vi "ADIS16448 IMU Calibration.vi"() -> ()   [LabVIEW 2015]
uses:
  <vilib>/Rock Robotics/SystemInterfaces/spilib/spi_bus.ctl
  <vilib>/Rock Robotics/WPI/SPI/WPI_SPIDevRef.ctl
  ADI MXP IMU/WPI_IMU_ADIS16448_Registers.ctl
  ADI MXP IMU/FRC_ADIS16448_IMU.lvlib
panel:
  out "Offset Registers":T1 {"zGYRO_OFF" format="%x"; "yGYRO_OFF" format="%x"; "xGYRO_OFF" format="%x"}
  out "Write Successful?":bool
  out "Timer":i32
  out "Device Found":bool
  # "FRC Analog Devices ADIS16448 IMU\nOffset Calibration Program"
  # "Instructions: \n* Place your robot in a stable location where it will not be bumped or moved.\n* Make sure that the IMU is securely mounted to the RoboRIO! \n* When ready, start the VI. The program will enable averaging inside of the IMU and will calculate the bias offset. \n* After recording data, the VI will save the data within the sensor for future use. \n* Running this utility again will overwrite the bias correction ."
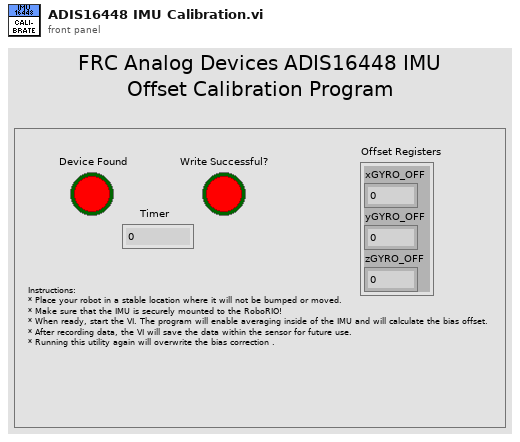
[diagram p1: front panel]
types:
  T1 = cluster{"xGYRO_OFF":u16, "yGYRO_OFF":u16, "zGYRO_OFF":u16}
  T2 = typedef "WPI_SPIDevRef.ctl" = cluster{"DevStatus":errorcluster, "Handle":i32, "SPI Bus":T3}
  T3 = typedef "spi_bus.ctl" = enum16{"SPI On-Board, CS0", "SPI On-Board, CS1", "SPI On-Board, CS2", "SPI On-Board, CS3", "SPI MXP", "Invalid"}
  T4 = typedef "FRC_ADIS16448_IMU.lvlib/WPI_IMU_ADIS16448_InterruptDevRef.ctl" = cluster{"ADI IMU DevRef":T5, "InterruptRef":T6}
  T5 = typedef "FRC_ADIS16448_IMU.lvlib/WPI_IMU_ADIS16448_IMUDevRef.ctl" = cluster{"DevStatus":errorcluster, "Handle":i32, "SPI Bus":T3, "Device Found":bool, "Device Ready":bool, "Yaw Axis":enum16{"X", "Y", "Z"}, "AHRS Algorithm":enum16{"Complementary", "Madgwick"}, "Serial":u16, "Lot ID 2":u16, "Lot ID 1":u16, "Product ID":u16}
  T6 = typedef "WPI_InterruptRef.ctl" = cluster{"DevStatus":errorcluster, "InterruptIndex":T7}
  T7 = typedef "FPGA_InterruptIndex.ctl" = enum8{"0", "1", "2", "3", "4", "5", "6", "7", "Invalid"}
  T8 = typedef "FRC_ADIS16448_IMU.lvlib/WPI_IMU_ADIS16448_Registers.ctl" = u8
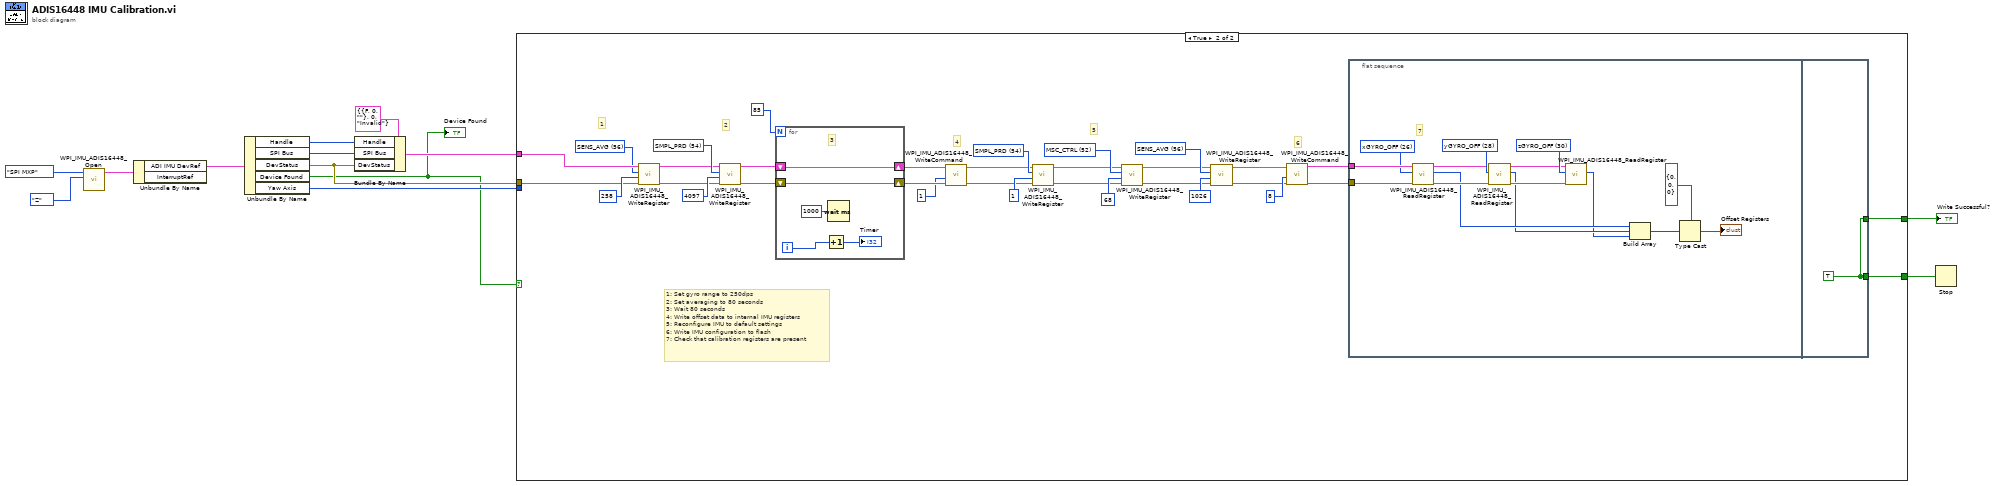
[diagram p0: block diagram]
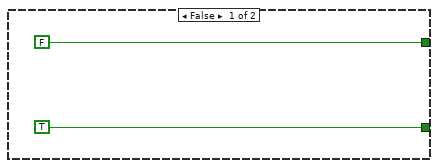
[diagram p2: hidden frame]
diagram:
  n1 = call "WPI_IMU_ADIS16448_Open.vi"("Yaw Axis"=enum16{"X", "Y", "Z"}."Z" ("Z Axis"), "SPI Chip Select"=spi_bus."SPI MXP") -> ("ADI IMU Interrupt DevRef"=w8:T4)  [unwired: 8 in, 1 out]
  n2 = Unbundle By Name(w8) -> ("ADI IMU DevRef"=w9:T5)  [unwired: 1 out]
  n3 = Unbundle By Name(w9) -> ("Handle"=w11:i32, "SPI Bus"=w10:T3, "DevStatus"=w5:errorcluster, "Device Found"=w1:bool, "Yaw Axis"=w6:enum16{"X", "Y", "Z"})
  "Device Found" <- w1
  n4 = Bundle By Name(cluster=T2 {"DevStatus"={"status"=FALSE, "code"=0, "source"=""}, "Handle"=0, "SPI Bus"=enum."Invalid"} ("SPIDevRef out"), "Handle"=w11, "SPI Bus"=w10, "DevStatus"=w5) -> (w7:T2)
  n5 = case shown="True" w1 {
    tunnel: w7 -> [_ w48]
    tunnel: w6 -> [_ _]
    tunnel: w5 -> [_ w45]
    tunnel: [TRUE w29] -> w3
    tunnel: [FALSE w16] -> w2
    frame False {
    }
    frame True {
      w32 = T8 56 items=["GLOB_CMD"=62, "SEQ_CNT"=58, "SMPL_PRD"=54, "SENS_AVG"=56, "MSC_CTRL"=52, "ERROR_FLAGS"=60, "TEMP"=44, "BARO"=40, "Z_MAG"=36, "Y_MAG"=32, "X_MAG"=28, "Z_ACCEL"=24, "Y_ACCEL"=20, "X_ACCEL"=16, "Z_GYRO"=12, "Y_GYRO"=8, "X_GYRO"=4, "PROD_ID"=86, "LOT_ID2"=84, "LOT_ID1"=82, "SERIAL_NUM"=88] ("ADIS16448 Register")
      w33 = T8 52 items=["GLOB_CMD"=62, "SEQ_CNT"=58, "SMPL_PRD"=54, "SENS_AVG"=56, "MSC_CTRL"=52, "ERROR_FLAGS"=60, "TEMP"=44, "BARO"=40, "Z_MAG"=36, "Y_MAG"=32, "X_MAG"=28, "Z_ACCEL"=24, "Y_ACCEL"=20, "X_ACCEL"=16, "Z_GYRO"=12, "Y_GYRO"=8, "X_GYRO"=4, "PROD_ID"=86, "LOT_ID2"=84, "LOT_ID1"=82, "SERIAL_NUM"=88] ("ADIS16448 Register")
      w31 = T8 54 items=["GLOB_CMD"=62, "SEQ_CNT"=58, "SMPL_PRD"=54, "SENS_AVG"=56, "MSC_CTRL"=52, "ERROR_FLAGS"=60, "TEMP"=44, "BARO"=40, "Z_MAG"=36, "Y_MAG"=32, "X_MAG"=28, "Z_ACCEL"=24, "Y_ACCEL"=20, "X_ACCEL"=16, "Z_GYRO"=12, "Y_GYRO"=8, "X_GYRO"=4, "PROD_ID"=86, "LOT_ID2"=84, "LOT_ID1"=82, "SERIAL_NUM"=88] ("ADIS16448 Register")
      w44 = T8 54 items=["GLOB_CMD"=62, "SEQ_CNT"=58, "SMPL_PRD"=54, "SENS_AVG"=56, "MSC_CTRL"=52, "ERROR_FLAGS"=60, "TEMP"=44, "BARO"=40, "Z_MAG"=36, "Y_MAG"=32, "X_MAG"=28, "Z_ACCEL"=24, "Y_ACCEL"=20, "X_ACCEL"=16, "Z_GYRO"=12, "Y_GYRO"=8, "X_GYRO"=4, "PROD_ID"=86, "LOT_ID2"=84, "LOT_ID1"=82, "SERIAL_NUM"=88] ("ADIS16448 Register")
      w47 = T8 56 items=["GLOB_CMD"=62, "SEQ_CNT"=58, "SMPL_PRD"=54, "SENS_AVG"=56, "MSC_CTRL"=52, "ERROR_FLAGS"=60, "TEMP"=44, "BARO"=40, "Z_MAG"=36, "Y_MAG"=32, "X_MAG"=28, "Z_ACCEL"=24, "Y_ACCEL"=20, "X_ACCEL"=16, "Z_GYRO"=12, "Y_GYRO"=8, "X_GYRO"=4, "PROD_ID"=86, "LOT_ID2"=84, "LOT_ID1"=82, "SERIAL_NUM"=88] ("ADIS16448 Register")
      # "5"
      # "6"
      # "4"
      # "2"
      # "1"
      # "1: Set gyro range to 250dps\n2: Set averaging to 80 seconds\n3: Wait 80 seconds\n4: Write offset data to internal IMU registers\n5: Reconfigure IMU to default settings\n6: Write IMU configuration to flash\n7: Check that calibration registers are present"
      n6 = call "WPI_IMU_ADIS16448_WriteRegister.vi"("error in (no error)"=w45, "Data"=u16 258, "ADIS16448 Register"=w47, "SPIDevRef in"=w48) -> ("error out"=w27:errorcluster, "SPIDevRef out"=w28:T2)  [unwired: 6 in]
      n7 = call "WPI_IMU_ADIS16448_WriteRegister.vi"("error in (no error)"=w27, "Data"=u16 4097, "ADIS16448 Register"=w44, "SPIDevRef in"=w28) -> ("error out"=w40:errorcluster, "SPIDevRef out"=w41:T2)  [unwired: 6 in]
      n8 = for {
        N: 85 -> [_]
        shift-right: [w68] -> w39
        shift-left: w41 -> [w68]
        shift-right: [w67] -> w38
        shift-left: w40 -> [w67]
        i -> [w65]
        # "3"
        n9 = Increment(x=w65) -> (x+1=→"Timer":i32)
        n10 = Wait (ms)(milliseconds to wait=u32 1000) -> ()  [unwired: 1 out]
      }
      n11 = call "WPI_IMU_ADIS16448_WriteCommand.vi"("error in (no error)"=w38, "Data"=u16 1, "SPIDevRef in"=w39) -> ("error out"=w25:errorcluster, "SPIDevRef out"=w26:T2)  [unwired: 7 in]
      n12 = call "WPI_IMU_ADIS16448_WriteRegister.vi"("error in (no error)"=w25, "Data"=u16 1, "ADIS16448 Register"=w31, "SPIDevRef in"=w26) -> ("error out"=w21:errorcluster, "SPIDevRef out"=w22:T2)  [unwired: 6 in]
      n13 = call "WPI_IMU_ADIS16448_WriteRegister.vi"("error in (no error)"=w21, "Data"=u16 68, "ADIS16448 Register"=w33, "SPIDevRef in"=w22) -> ("error out"=w23:errorcluster, "SPIDevRef out"=w24:T2)  [unwired: 6 in]
      n14 = call "WPI_IMU_ADIS16448_WriteRegister.vi"("error in (no error)"=w23, "Data"=u16 1026, "ADIS16448 Register"=w32, "SPIDevRef in"=w24) -> ("error out"=w19:errorcluster, "SPIDevRef out"=w20:T2)  [unwired: 6 in]
      n15 = call "WPI_IMU_ADIS16448_WriteCommand.vi"("error in (no error)"=w19, "Data"=u16 8, "SPIDevRef in"=w20) -> ("error out"=w17:errorcluster, "SPIDevRef out"=w18:T2)  [unwired: 7 in]
      n16 = flat-sequence {
        tunnel: w18 -> [w63]
        tunnel: w17 -> [w62]
        tunnel: [w64] -> w29
        tunnel: [w64] -> w16
        frame #0 {
          w59 = T8 30 items=["zGYRO_OFF"=30, "yGYRO_OFF"=28, "xGYRO_OFF"=26, "GLOB_CMD"=62, "SEQ_CNT"=58, "SMPL_PRD"=54, "SENS_AVG"=56, "MSC_CTRL"=52, "zACCEL_OFF"=36, "yACCEL_OFF"=34, "xACCEL_OFF"=32, "ERROR_FLAGS"=60, "TEMP"=24, "BARO"=22, "Z_MAG"=20, "Y_MAG"=18, "X_MAG"=16, "Z_ACCEL"=14, "Y_ACCEL"=12, "X_ACCEL"=10, "Z_GYRO"=8, "Y_GYRO"=6, "X_GYRO"=4, "PROD_ID"=86, "LOT_ID2"=84, "LOT_ID1"=82, "SERIAL_NUM"=88] ("ADIS16448 Register")
          w60 = T8 28 items=["zGYRO_OFF"=30, "yGYRO_OFF"=28, "xGYRO_OFF"=26, "GLOB_CMD"=62, "SEQ_CNT"=58, "SMPL_PRD"=54, "SENS_AVG"=56, "MSC_CTRL"=52, "zACCEL_OFF"=36, "yACCEL_OFF"=34, "xACCEL_OFF"=32, "ERROR_FLAGS"=60, "TEMP"=24, "BARO"=22, "Z_MAG"=20, "Y_MAG"=18, "X_MAG"=16, "Z_ACCEL"=14, "Y_ACCEL"=12, "X_ACCEL"=10, "Z_GYRO"=8, "Y_GYRO"=6, "X_GYRO"=4, "PROD_ID"=86, "LOT_ID2"=84, "LOT_ID1"=82, "SERIAL_NUM"=88] ("ADIS16448 Register")
          w61 = T8 26 items=["zGYRO_OFF"=30, "yGYRO_OFF"=28, "xGYRO_OFF"=26, "GLOB_CMD"=62, "SEQ_CNT"=58, "SMPL_PRD"=54, "SENS_AVG"=56, "MSC_CTRL"=52, "zACCEL_OFF"=36, "yACCEL_OFF"=34, "xACCEL_OFF"=32, "ERROR_FLAGS"=60, "TEMP"=24, "BARO"=22, "Z_MAG"=20, "Y_MAG"=18, "X_MAG"=16, "Z_ACCEL"=14, "Y_ACCEL"=12, "X_ACCEL"=10, "Z_GYRO"=8, "Y_GYRO"=6, "X_GYRO"=4, "PROD_ID"=86, "LOT_ID2"=84, "LOT_ID1"=82, "SERIAL_NUM"=88] ("ADIS16448 Register")
          # "7"
          n17 = call "WPI_IMU_ADIS16448_ReadRegister.vi"("error in (no error)"=w62, "ADIS16448 Register"=w61, "SPIDevRef in"=w63) -> ("error out"=w57:errorcluster, "Register Value"=w54:u16, "SPIDevRef out"=w58:T2)  [unwired: 6 in]
          n18 = call "WPI_IMU_ADIS16448_ReadRegister.vi"("error in (no error)"=w57, "ADIS16448 Register"=w60, "SPIDevRef in"=w58) -> ("error out"=w55:errorcluster, "Register Value"=w53:u16, "SPIDevRef out"=w56:T2)  [unwired: 6 in]
          n19 = call "WPI_IMU_ADIS16448_ReadRegister.vi"("error in (no error)"=w55, "ADIS16448 Register"=w59, "SPIDevRef in"=w56) -> ("Register Value"=w52:u16)  [unwired: 6 in, 2 out]
          n20 = Build Array(w54, w53, w52) -> (w51:u16[])
          n21 = Type Cast(type=T1 {"xGYRO_OFF"=0, "yGYRO_OFF"=0, "zGYRO_OFF"=0} ("Offset Registers 2"), x=w51) -> (*(type *) &x=→"Offset Registers":T1)
        }
        frame #1 {
          w64 = TRUE
        }
      }
    }
  }
  "Write Successful?" <- w2
  n22 = Stop(stop? (T)=w3) -> ()
